vi "matlab_TI2_filter.vi"(8 "error in":errorcluster, 10 "Filter":u16(ring) items=["1-", "2-", "3-", "4-", "5-", "6-"]) -> (0 "error out":errorcluster)   [LabVIEW 2018]
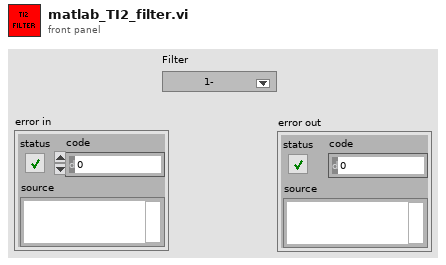
[diagram p1: front panel]
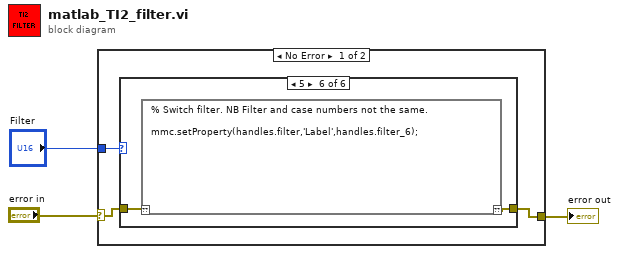
[diagram p0: block diagram]
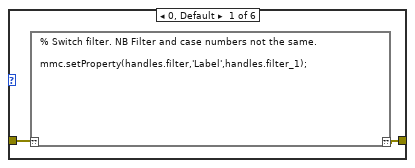
[diagram p2: hidden frame]
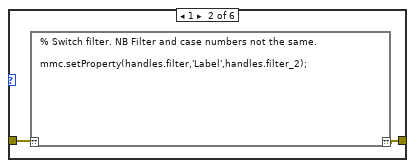
[diagram p3: hidden frame]
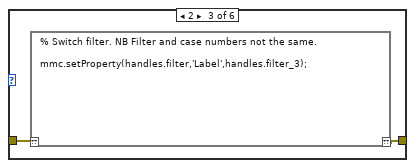
[diagram p4: hidden frame]
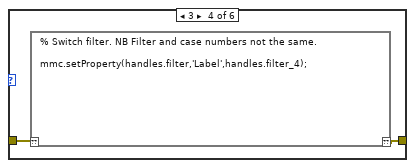
[diagram p5: hidden frame]
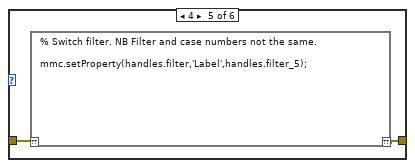
[diagram p6: hidden frame]
diagram:
  n1 = case shown="No Error" "error in" {
    selector: "error in" -> [w5 w19]
    tunnel: [w4 w19] -> w2
    tunnel: "Filter" -> [w6 _]
    frame No Error {
      n2 = case shown="5" w6 {
        tunnel: w5 -> [w8 w10 w12 w14 w16 w18]
        tunnel: [w7 w9 w11 w13 w15 w17] -> w4
        frame 0, Default {
          n3 = script code="% Switch filter. NB Filter and case numbers not the same.\n\nmmc.setProperty(handles.filter,'Label',handles.filter_1);"("??"=w8) -> ("??"=w7:errorcluster)
        }
        frame 1 {
          n4 = script code="% Switch filter. NB Filter and case numbers not the same.\n\nmmc.setProperty(handles.filter,'Label',handles.filter_2);"("??"=w10) -> ("??"=w9:errorcluster)
        }
        frame 2 {
          n5 = script code="% Switch filter. NB Filter and case numbers not the same.\n\nmmc.setProperty(handles.filter,'Label',handles.filter_3);"("??"=w12) -> ("??"=w11:errorcluster)
        }
        frame 3 {
          n6 = script code="% Switch filter. NB Filter and case numbers not the same.\n\nmmc.setProperty(handles.filter,'Label',handles.filter_4);"("??"=w14) -> ("??"=w13:errorcluster)
        }
        frame 4 {
          n7 = script code="% Switch filter. NB Filter and case numbers not the same.\n\nmmc.setProperty(handles.filter,'Label',handles.filter_5);"("??"=w16) -> ("??"=w15:errorcluster)
        }
        frame 5 {
          n8 = script code="% Switch filter. NB Filter and case numbers not the same.\n\nmmc.setProperty(handles.filter,'Label',handles.filter_6);"("??"=w18) -> ("??"=w17:errorcluster)
        }
      }
    }
    frame Error {
    }
  }
  "error out" <- w2
